vi "Ne4lr.vi"() -> ()   [LabVIEW 2012]
uses:
  <vilib>/Analysis/NI_AALBase.lvlib
  <vilib>/Analysis/NI_AALPro.lvlib
panel:
  in  "Noise amplitude":dbl(knob) scale=0.0..3.0
  in  "stop":bool
  in  "Noise":u16(ring) items=["Periodic Random", "Uniform white", "Gaussian white"]
  in  "Sine frequency":dbl(slide) scale=0.1..1.0
  in  "Slide":dbl(slide) scale=100.0..1000.0
  out "Waveform Graph":dbl[](graph)
  in  "Square wave duty cycle(%)":dbl
  in  "Samples":i32
  in  "Signal Type":enum16{"sine", "square"}(ring)
  in  "Frequency":dbl(knob) scale=0.1..100.0
  in  "Signal amplitude":dbl(slide) scale=1.0..10.0
  in  "Out":bool
  # "Radio imp"
  # "Video imp"
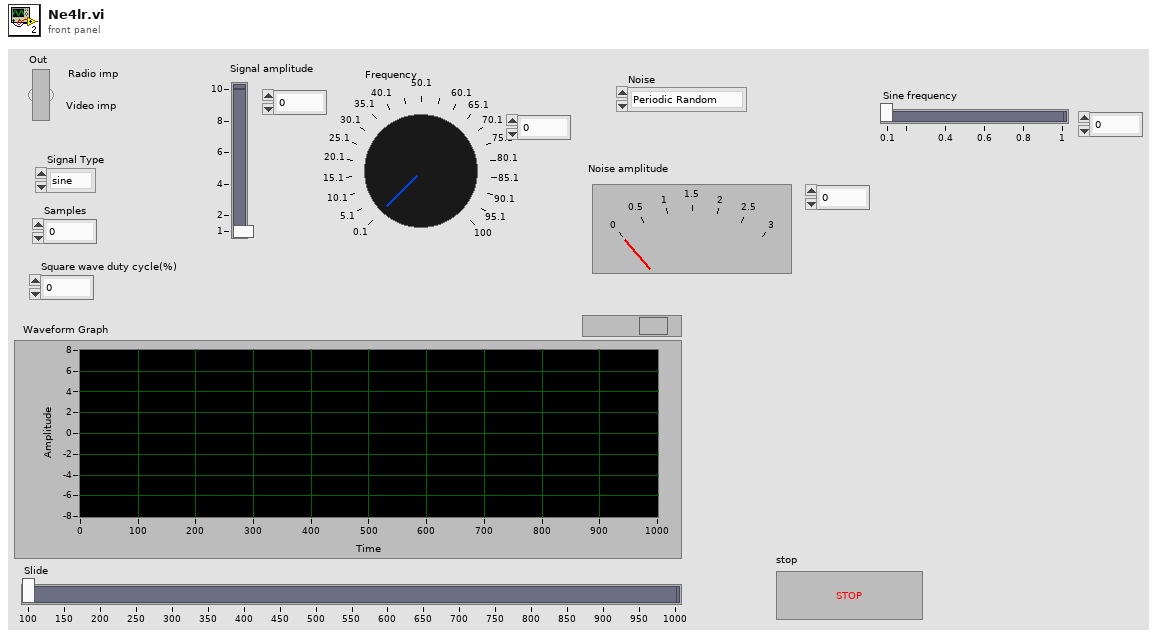
[diagram p1: front panel]
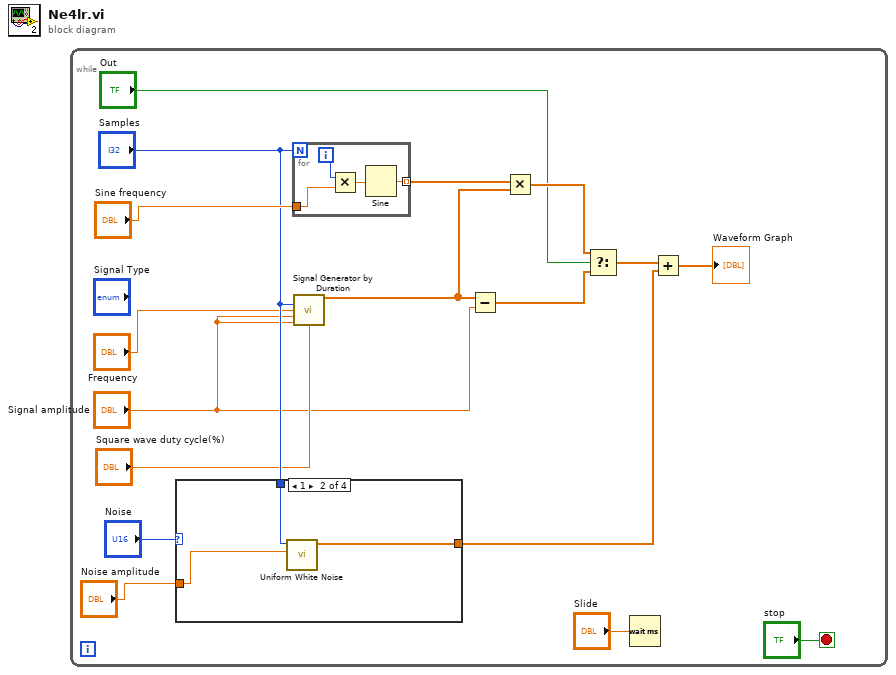
[diagram p0: block diagram]
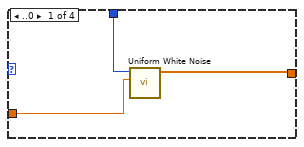
[diagram p2: hidden frame]
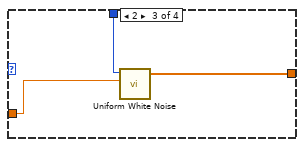
[diagram p3: hidden frame]
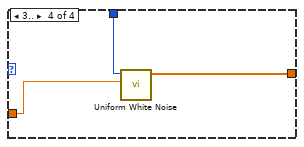
[diagram p4: hidden frame]
diagram:
  n1 = while {
    stop <- "stop" stop-if-true
    n2 = case shown="1" "Noise" {
      tunnel: "Samples" -> [w19 w23 w25 w28]
      tunnel: [w20 w22 w26 w29] -> w5
      tunnel: "Noise amplitude" -> [w18 w21 w24 w27]
      frame ..0 {
        n3 = call <vilib>:"Uniform White Noise.vi"("amplitude"=w18, "samples"=w19) -> ("uniform white noise"=w20:dbl[])  [unwired: 8 in, 1 out]
      }
      frame 1 {
        n4 = call <vilib>:"Uniform White Noise.vi"("amplitude"=w21, "samples"=w23) -> ("uniform white noise"=w22:dbl[])  [unwired: 8 in, 1 out]
      }
      frame 2 {
        n5 = call <vilib>:"Uniform White Noise.vi"("amplitude"=w24, "samples"=w25) -> ("uniform white noise"=w26:dbl[])  [unwired: 8 in, 1 out]
      }
      frame 3.. {
        n6 = call <vilib>:"Uniform White Noise.vi"("amplitude"=w27, "samples"=w28) -> ("uniform white noise"=w29:dbl[])  [unwired: 8 in, 1 out]
      }
    }
    n7 = for {
      N: "Samples" -> [_]
      tunnel: "Sine frequency" -> [w31]
      tunnel: [w30] -> w11 mode=indexing
      i -> [w32]
      n8 = Multiply(x=w32, y=w31) -> (x*y=w33:dbl)
      n9 = Sine(x=w33) -> (sin(x)=w30:dbl)
    }
    n10 = call <vilib>:"Signal Generator by Duration.vi"("# of samples"="Samples", "frequency"="Frequency", "amplitude"="Signal amplitude", "dc offset"="Signal amplitude", "square wave duty cycle (%)"="Square wave duty cycle(%)") -> ("signal"=w10:dbl[])  [unwired: 7 in, 3 out]
    n11 = Subtract(x=w10, y="Signal amplitude") -> (x-y=w9:dbl[])
    n12 = Multiply(x=w11, y=w10) -> (x*y=w8:dbl[])
    n13 = Select(t=w8, s="Out", f=w9) -> (s? t:f=w6:dbl[])
    n14 = Wait (ms)(milliseconds to wait="Slide") -> ()  [unwired: 1 out]
    n15 = Add(x=w6, y=w5) -> (x+y=→"Waveform Graph":dbl[])
  }
